vi "Test Comm Multi.vi"() -> ()   [LabVIEW 2021]
uses:
  ChannelCommon/typedef/FIFO Config.ctl
  ChannelCommon/ChannelCommon.lvlib
  CIFChannels/Typedef/Direction.ctl
  CIFChannels/CIFChannels.lvclass
  ChannelCommon/typedef/TimeStamps.ctl
  FIFO_U8_Multi/CIF_Fifo_U8_Multi.lvclass
  ChannelCommon/typedef/New FIFO Instance Configuration.ctl
  FIFO_U8/CIF_NIChn_Fifo_U8.lvclass
  D:/dev/Packages/Channel_Manager/src/CIF_NIChn/FIFO_U8/CIF_NIChn_Fifo_U8.lvclass
  D:/dev/Packages/Channel_Manager/src/CIF_NIChn/NIChn/CIF_NIChn.lvclass
  D:/dev/Packages/Channel_Manager/src/CIFChannels/CIFChannels.lvclass
  D:/dev/Packages/Channel_Manager/src/CIF_NIChn/FIFO_U8_Multi/CIF_Fifo_U8_Multi.lvclass
  CIF_Fifo_Raw.lvclass
  D:/dev/Packages/Channel_Manager/src/CIF_NIChn/FIFO_RAW_Multi/CIF_Fifo_Raw.lvclass
panel:
  out "status":string
  out "pass":bool
  out "error out":errorcluster
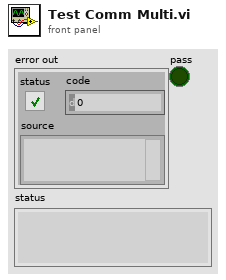
[diagram p1: front panel]
types:
  T1 = typedef "CIFChannels.lvclass/Direction.ctl" = enum16{"Publisher", "Subscriber"}
  T2 = typedef "ChannelCommon.lvlib/New FIFO Instance Configuration.ctl" = cluster{"Primary":bool, "Backpressure":bool, "Message/FIFO Override":u32}
  T3 = typedef "ChannelCommon.lvlib/TimeStamps.ctl" = cluster{"ClockID":u8, "T0":i64, "T_Out":i64}
  T4 = typedef "ChannelCommon.lvlib/FIFO Config.ctl" = cluster{"Max Bytes/Msg":u64, "Max Msg/FIFO":u64, "Flags":u64}
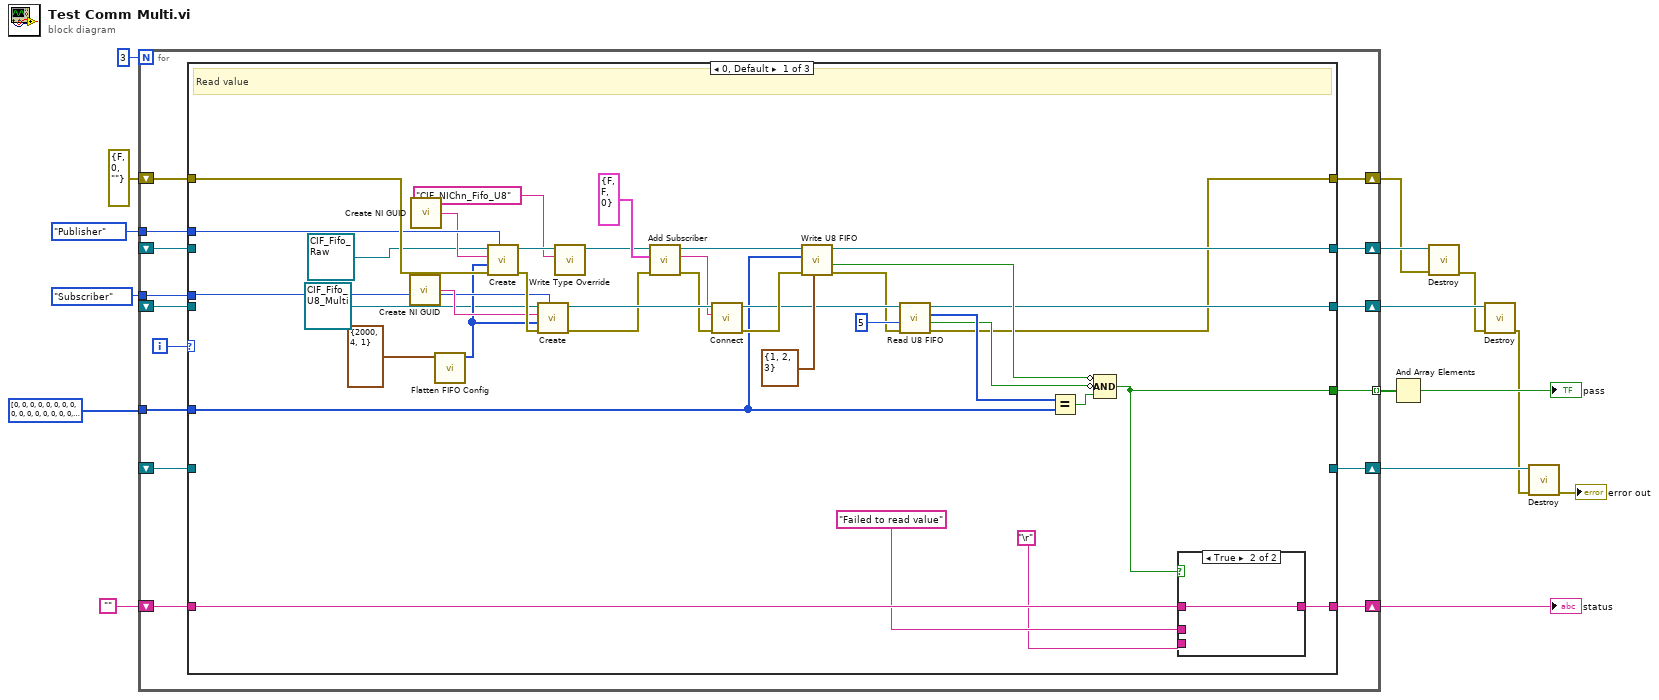
[diagram p0: block diagram]
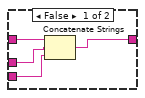
[diagram p2: hidden frame]
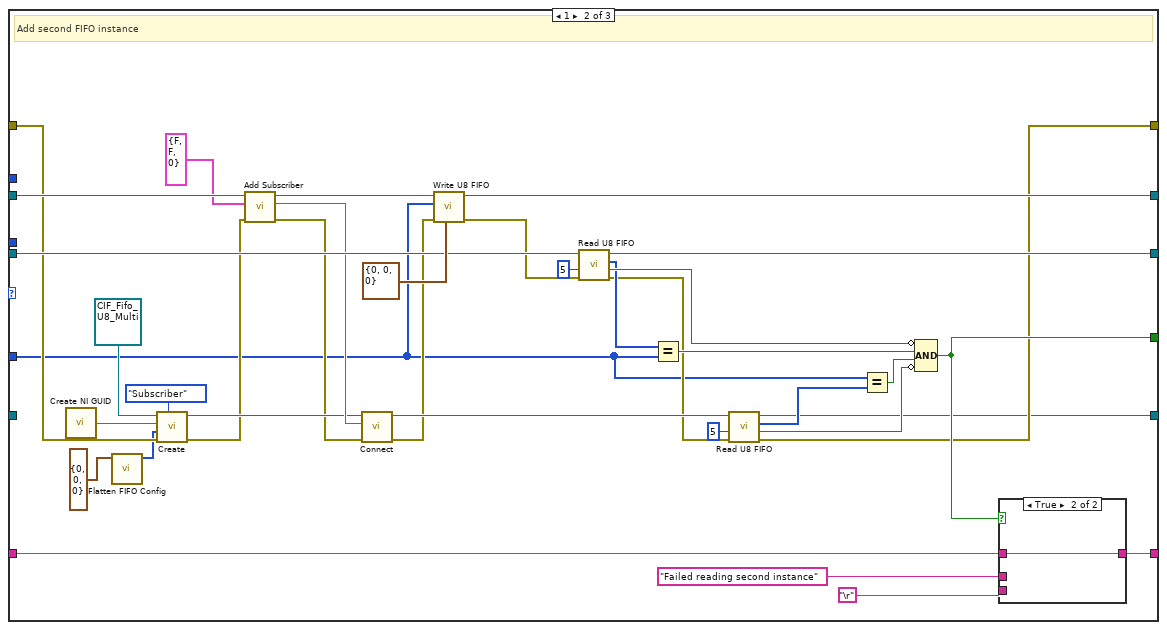
[diagram p3: hidden frame]
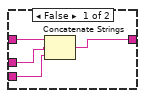
[diagram p4: hidden frame]
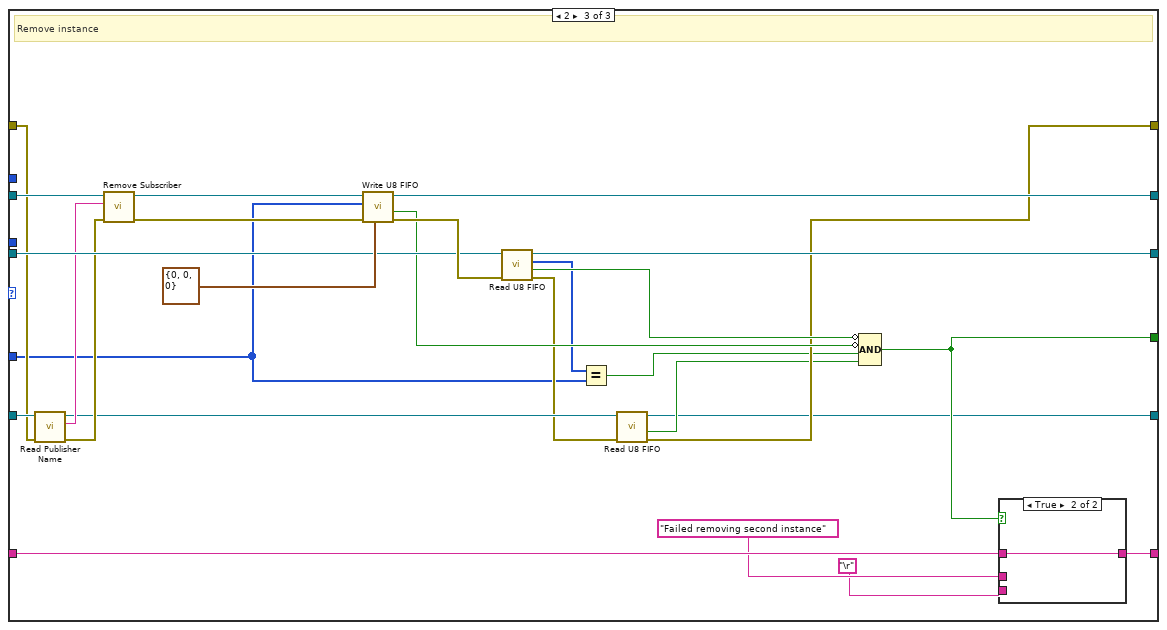
[diagram p5: hidden frame]
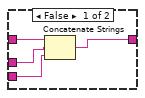
[diagram p6: hidden frame]
diagram:
  n1 = for {
    N: 3 -> [_]
    tunnel: [w31] -> w16 mode=indexing
    shift-right: [w22] -> w6
    shift-left: errorcluster {"status"=FALSE, "code"=0, "source"=""} ("error out") -> [w30]
    shift-right: [w27] -> w12
    shift-left: "" -> [w28]
    tunnel: Direction."Subscriber" ("Direction") -> [w26]
    tunnel: Direction."Publisher" ("Direction") -> [w25]
    shift-right: [w24] -> w8
    shift-left: _ -> [w20]
    shift-right: [w23] -> w7
    shift-left: _ -> [w21]
    tunnel: u8[] [0, 0, 0, 0, 0, 0, 0, 0, 0, 0, 0, 0, 0, 0, 0, 0, 0, 0, 0, 0, 0, 0, 0, 0, 0, 0, 0, 0, 0, 0, 0, 0, 0, 0, 0, 0, 0, 0, 0, 0, 0, 0, 0, 0, 0, 0, 0, 0, 0, 0, 0, 0, 0, 0, 0, 0, 0, 0, 0, 0, 0, 0, 0, 0, 0, 0, 0, 0, 0, 0, 0, 0, 0, 0, 0, 0, 0, 0, 0, 0, 0, 0, 0, 0, 0, 0, 0, 0, 0, 0, 0, 0, 0, 0, 0, 0, 0, 0, 0, 0, 0, 0, 0, 0, 0, 0, 0, 0, 0, 0, 0, 0, 0, 0, 0, 0, 0, 0, 0, 0, 0, 0, 0, 0, 0, 0, 0, 0, 0, 0, 0, 0, 0, 0, 0, 0, 0, 0, 0, 0, 0, 0, 0, 0, 0, 0, 0, 0, 0, 0, 0, 0, 0, 0, 0, 0, 0, 0, 0, 0, 0, 0, 0, 0, 0, 0, 0, 0, 0, 0, 0, 0, 0, 0, 0, 0, 0, 0, 0, 0, 0, 0, 0, 0, 0, 0, 0, 0, 0, 0, 0, 0, 0, 0, 0, 0, 0, 0, 0, 0, 0, 0, 0, 0, 0, 0, 0, 0, 0, 0, 0, 0, 0, 0, 0, 0, 0, 0, 0, 0, 0, 0, 0, 0, 0, 0, 0, 0, 0, 0, 0, 0, 0, 0, 0, 0, 0, 0, 0, 0, 0, 0, 0, 0, 0, 0, 0, 0, 0, 0, 0, 0, 0, 0, 0, 0, 0, 0, 0, 0, 0, 0, 0, 0, 0, 0, 0, 0, 0, 0, 0, 0, 0, 0, 0, 0, 0, 0, 0, 0, 0, 0, 0, 0, 0, 0, 0, 0, 0, 0, 0, 0, 0, 0, 0, 0, 0, 0, 0, 0, 0, 0, 0, 0, 0, 0, 0, 0, 0, 0, 0, 0, 0, 0, 0, 0, 0, 0, 0, 0, 0, 0, 0, 0, 0, 0, 0, 0, 0, 0, 0, 0, 0, 0, 0, 0, 0, 0, 0, 0, 0, 0, 0, 0, 0, 0, 0, 0, 0, 0, 0, 0, 0, 0, 0, 0, 0, 0, 0, 0, 0, 0, 0, 0, 0, 0, 0, 0, 0, 0, 0, 0, 0, 0, 0, 0, 0, 0, 0, 0, 0, 0, 0, 0, 0, 0, 0, 0, 0, 0, 0, 0, 0, 0, 0, 0, 0, 0, 0, 0, 0, 0, 0, 0, 0, 0, 0, 0, 0, 0, 0, 0, 0, 0, 0, 0, 0, 0, 0, 0, 0, 0, 0, 0, 0, 0, 0, 0, 0, 0, 0, 0, 0, 0, 0, 0, 0, 0, 0, 0, 0, 0, 0, 0, 0, 0, 0, 0, 0, 0, 0, 0, 0, 0, 0, 0, 0, 0, 0, 0, 0, 0, 0, 0, 0, 0, 0, 0, 0, 0, 0, 0, 0, 0, 0, 0, 0, 0, 0, 0, 0, 0, 0, 0, 0, 0, 0, 0, 0, 0, 0, 0, 0, 0, 0, 0, 0, 0, 0, 0, 0, 0, 0, 0, 0, 0, 0, 0, 0, 0, 0, 0, 0, 0, 0, 0, 0, 0, 0, 0, 0, 0, 0, 0, 0, 0, 0, 0, 0, 0, 0, 0, 0, 0, 0, 0, 0, 0, 0, 0, 0, 0, 0, 0, 0, 0, 0, 0, 0, 0, 0, 0, 0, 0, 0, 0, 0, 0, 0, 0, 0, 0, 0, 0, 0, 0, 0, 0, 0, 0, 0, 0, 0, 0, 0, 0, 0, 0, 0, 0, 0, 0, 0, 0, 0, 0, 0, 0, 0, 0, 0, 0, 0, 0, 0, 0, 0, 0, 0, 0, 0, 0, 0, 0, 0, 0, 0, 0, 0, 0, 0, 0, 0, 0, 0, 0, 0, 0, 0, 0, 0, 0, 0, 0, 0, 0, 0, 0, 0, 0, 0, 0, 0, 0, 0, 0, 0, 0, 0, 0, 0, 0, 0, 0, 0, 0, 0, 0, 0, 0, 0, 0, 0, 0, 0, 0, 0, 0, 0, 0, 0, 0, 0, 0, 0, 0, 0, 0, 0, 0, 0, 0, 0, 0, 0, 0, 0, 0, 0, 0, 0, 0, 0, 0, 0, 0, 0, 0, 0, 0, 0, 0, 0, 0, 0, 0, 0, 0, 0, 0, 0, 0, 0, 0, 0, 0, 0, 0, 0, 0, 0, 0, 0, 0, 0, 0, 0, 0, 0, 0, 0, 0, 0, 0, 0, 0, 0, 0, 0, 0, 0, 0, 0, 0, 0, 0, 0, 0, 0, 0, 0, 0, 0, 0, 0, 0, 0, 0, 0, 0, 0, 0, 0, 0, 0, 0, 0, 0, 0, 0, 0, 0, 0, 0, 0, 0, 0, 0, 0, 0, 0, 0, 0, 0, 0, 0, 0, 0, 0, 0, 0, 0, 0, 0, 0, 0, 0, 0, 0, 0, 0, 0, 0, 0, 0, 0, 0, 0, 0, 0, 0, 0, 0, 0, 0, 0, 0, 0, 0, 0, 0, 0, 0, 0, 0, 0, 0, 0, 0, 0, 0, 0, 0, 0, 0, 0, 0, 0, 0, 0, 0, 0, 0, 0, 0, 0, 0, 0, 0, 0, 0, 0, 0, 0, 0, 0, 0, 0, 0, 0, 0, 0, 0, 0, 0, 0, 0, 0, 0, 0, 0, 0, 0, 0, 0, 0, 0, 0, 0, 0, 0, 0, 0, 0, 0, 0, 0, 0, 0, 0, 0, 0, 0, 0, 0, 0, 0, 0, 0, 0, 0, 0, 0, 0, 0, 0, 0, 0, 0, 0, 0, 0, 0, 0, 0, 0, 0, 0, 0, 0, 0, 0, 0, 0, 0, 0, 0, 0, 0, 0, 0, 0, 0, 0, 0, 0, 0, 0, 0, 0, 0, 0, 0, 0, 0, 0, 0, 0, 0, 0, 0, 0, 0, 0, 0, 0, 0, 0, 0, 0, 0, 0, 0, 0, 0, 0, 0, 0, 0, 0, 0, 0, 0, 0, 0, 0, 0, 0, 0, 0, 0, 0, 0, 0, 0, 0, 0, 0, 0, 0, 0, 0, 0, 0, 0, 0, 0, 0, 0, 0, 0, 0, 0, 0, 0, 0, 0, 0, 0, 0, 1] ("Data in") -> [w19]
    shift-right: [w17] -> w4
    shift-left: _ -> [w18]
    i -> [w29]
    n2 = case shown="0, Default" w29 {
      tunnel: [w63 w106 w136] -> w31
      tunnel: w30 -> [w61 w89 w129]
      tunnel: [w44 w79 w121] -> w22
      tunnel: w28 -> [w68 w110 w142]
      tunnel: [w67 w109 w141] -> w27
      tunnel: w26 -> [w59 _ _]
      tunnel: w25 -> [w58 _ _]
      tunnel: [w46 w80 w133] -> w24
      tunnel: [w51 w98 w124] -> w23
      tunnel: w21 -> [_ w97 w132]
      tunnel: w20 -> [_ w99 w134]
      tunnel: w19 -> [w37 w78 w117]
      tunnel: w18 -> [_ _ w130]
      tunnel: [_ w74 w116] -> w17
      frame 0, Default {
        # "Read value"
        n3 = call <vilib>:"Create NI GUID.vi"() -> ("NI GUID"=w60:string)
        n4 = call <vilib>:"Create NI GUID.vi"() -> ("NI GUID"=w56:string)
        n5 = call "Flatten FIFO Config.vi"("FIFO Config in"=T4 {"Max Bytes/Msg"=2000, "Max Msg/FIFO"=4, "Flags"=1}) -> ("Flattened FIFO Config"=w54:u8[])  [unwired: 10 in]
        n6 = call-dynamic "Create.vi"("Direction"=w58, "error in (no error)"=w61, "Custom Config Data"=w54, "Name"=w56, "CIF_Fifo_Raw_Multi in"=refnum<class "CIF_Fifo_Raw.lvclass"> refnum ("CIF_Fifo_Raw_Multi.lvclass")) -> ("error out"=w62:errorcluster, "CIF_Fifo_Raw_Multi out"=w34:refnum<class "CIF_Fifo_Raw.lvclass">)  [unwired: 5 in]
        n7 = call-dynamic "Create.vi"("Direction"=w59, "error in (no error)"=w62, "Custom Config Data"=w54, "Name"=w60, "CIF_Fifo_U8 in"=refnum<class "CIF_Fifo_U8_Multi.lvclass"> refnum ("CIF_DAQ_DVR_Multi.lvclass")) -> ("error out"=w40:errorcluster, "CIF_Fifo_U8 out"=w55:refnum<class "CIF_Fifo_U8_Multi.lvclass">)  [unwired: 5 in]
        n8 = call "Write Type Override.vi"("Type Override"="CIF_NIChn_Fifo_U8", "CIF_Fifo_Raw_Multi in"=w34) -> ("CIF_Fifo_Raw_Multi out"=w33:refnum<class "CIF_Fifo_Raw.lvclass">)  [unwired: 8 in, 1 out]
        n9 = call-dynamic "Add Subscriber.vi"("error in (no error)"=w40, "New FIFO Instance Config"=T2 {"Primary"=FALSE, "Backpressure"=FALSE, "Message/FIFO Override"=0}, "CIF_Fifo_Raw_Multi in"=w33) -> ("error out"=w39:errorcluster, "New Publisher"=w41:string, "CIF_Fifo_Raw_Multi out"=w42:refnum<class "CIF_Fifo_Raw.lvclass">)  [unwired: 6 in]
        n10 = call-dynamic "Connect.vi"("error in (no error)"=w39, "Connection Name"=w41, "CIFTag in"=w55) -> ("error out"=w53:errorcluster, "CIFTag out"=w49:refnum<class "CIF_Fifo_U8_Multi.lvclass">)  [unwired: 7 in]
        n11 = call-dynamic "Write U8 FIFO.vi"("FIFO Timestamps"=T3 {"ClockID"=1, "T0"=2, "T_Out"=3}, "error in (no error)"=w53, "Data in"=w37, "CIF_Fifo_U8 in"=w42) -> ("error out"=w36:errorcluster, "timed out?"=w50:bool, "CIF_Fifo_U8 out"=w51:refnum<class "CIF_Fifo_Raw.lvclass">)  [unwired: 4 in, 1 out]
        n12 = call-dynamic "Read U8 FIFO.vi"("error in (no error)"=w36, "Timeout (ms)"=5, "CIFFIFO in"=w49) -> ("error out"=w44:errorcluster, "timed out?"=w45:bool, "Data out"=w47:u8[], "CIFFIFO out"=w46:refnum<class "CIF_Fifo_U8_Multi.lvclass">)  [unwired: 4 in, 1 out]
        n13 = Equal?(x=w47, y=w37) -> (x = y?=w64:bool)
        n14 = Compound Arithmetic op=AND(invert w50, invert w45, w64) -> (w63:bool)
        n15 = case shown="True" w63 {
          tunnel: w68 -> [w72 w73]
          tunnel: [w69 w73] -> w67
          tunnel: "Failed to read value" -> [w71 _]
          tunnel: "\r" -> [w70 _]
          frame False {
            n16 = Concatenate Strings(w72, w71, w70) -> (w69:string)
          }
          frame True {
          }
        }
      }
      frame 1 {
        # "Add second FIFO instance"
        n17 = call <vilib>:"Create NI GUID.vi"() -> ("NI GUID"=w94:string)
        n18 = call "Flatten FIFO Config.vi"("FIFO Config in"=T4 {"Max Bytes/Msg"=0, "Max Msg/FIFO"=0, "Flags"=0}) -> ("Flattened FIFO Config"=w88:u8[])  [unwired: 10 in]
        n19 = call-dynamic "Create.vi"("Direction"=Direction."Subscriber", "error in (no error)"=w89, "Custom Config Data"=w88, "Name"=w94, "CIF_Fifo_U8 in"=refnum<class "CIF_Fifo_U8_Multi.lvclass"> refnum ("CIF_DAQ_DVR_Multi.lvclass")) -> ("error out"=w90:errorcluster, "CIF_Fifo_U8 out"=w92:refnum<class "CIF_Fifo_U8_Multi.lvclass">)  [unwired: 5 in]
        n20 = call-dynamic "Add Subscriber.vi"("error in (no error)"=w90, "New FIFO Instance Config"=T2 {"Primary"=FALSE, "Backpressure"=FALSE, "Message/FIFO Override"=0}, "CIF_Fifo_U8 in"=w97) -> ("error out"=w91:errorcluster, "New Publisher"=w93:string, "CIF_Fifo_U8 out"=w96:refnum<class "CIF_Fifo_U8_Multi.lvclass">)  [unwired: 6 in]
        n21 = call-dynamic "Connect.vi"("error in (no error)"=w91, "Connection Name"=w93, "CIFTag in"=w92) -> ("error out"=w83:errorcluster, "CIFTag out"=w84:refnum<class "CIF_Fifo_U8_Multi.lvclass">)  [unwired: 7 in]
        n22 = call-dynamic "Write U8 FIFO.vi"("FIFO Timestamps"=T3 {"ClockID"=0, "T0"=0, "T_Out"=0}, "error in (no error)"=w83, "Data in"=w78, "CIF_Fifo_U8 in"=w96) -> ("error out"=w77:errorcluster, "CIF_Fifo_U8 out"=w98:refnum<class "CIF_Fifo_U8_Multi.lvclass">)  [unwired: 4 in, 2 out]
        n23 = call-dynamic "Read U8 FIFO.vi"("error in (no error)"=w77, "Timeout (ms)"=5, "CIFFIFO in"=w99) -> ("error out"=w81:errorcluster, "timed out?"=w102:bool, "Data out"=w101:u8[], "CIFFIFO out"=w80:refnum<class "CIF_NIChn_Fifo_U8.lvclass">)  [unwired: 4 in, 1 out]
        n24 = Equal?(x=w101, y=w78) -> (x = y?=w104:bool)
        n25 = call-dynamic "Read U8 FIFO.vi"("error in (no error)"=w81, "Timeout (ms)"=5, "CIFFIFO in"=w84) -> ("error out"=w79:errorcluster, "timed out?"=w75:bool, "Data out"=w82:u8[], "CIFFIFO out"=w74:refnum<class "CIF_Fifo_U8_Multi.lvclass">)  [unwired: 4 in, 1 out]
        n26 = Equal?(x=w78, y=w82) -> (x = y?=w105:bool)
        n27 = Compound Arithmetic op=AND(invert w102, w104, w105, invert w75) -> (w106:bool)
        n28 = case shown="True" w106 {
          tunnel: w110 -> [w114 w115]
          tunnel: [w111 w115] -> w109
          tunnel: "Failed reading second instance" -> [w113 _]
          tunnel: "\r" -> [w112 _]
          frame False {
            n29 = Concatenate Strings(w114, w113, w112) -> (w111:string)
          }
          frame True {
          }
        }
      }
      frame 2 {
        # "Remove instance"
        n30 = call "Read Publisher Name.vi"("error in (no error)"=w129, "CIFChannels in"=w130) -> ("error out"=w126:errorcluster, "Publisher Name"=w128:string, "CIFChannels out"=w123:refnum<class "CIF_Fifo_U8_Multi.lvclass">)  [unwired: 7 in]
        n31 = call-dynamic "Remove Subscriber.vi"("error in (no error)"=w126, "Publisher to Remove"=w128, "CIF_Fifo_U8 in"=w132) -> ("error out"=w127:errorcluster, "CIF_Fifo_U8 out"=w131:refnum<class "CIF_Fifo_U8_Multi.lvclass">)  [unwired: 7 in]
        n32 = call-dynamic "Write U8 FIFO.vi"("FIFO Timestamps"=T3 {"ClockID"=0, "T0"=0, "T_Out"=0}, "error in (no error)"=w127, "Data in"=w117, "CIF_Fifo_U8 in"=w131) -> ("error out"=w138:errorcluster, "timed out?"=w125:bool, "CIF_Fifo_U8 out"=w124:refnum<class "CIF_Fifo_U8_Multi.lvclass">)  [unwired: 4 in, 1 out]
        n33 = call-dynamic "Read U8 FIFO.vi"("error in (no error)"=w138, "CIFFIFO in"=w134) -> ("error out"=w122:errorcluster, "timed out?"=w137:bool, "Data out"=w120:u8[], "CIFFIFO out"=w133:refnum<class "CIF_NIChn_Fifo_U8.lvclass">)  [unwired: 5 in, 1 out]
        n34 = Equal?(x=w120, y=w117) -> (x = y?=w119:bool)
        n35 = call-dynamic "Read U8 FIFO.vi"("error in (no error)"=w122, "CIFFIFO in"=w123) -> ("error out"=w121:errorcluster, "timed out?"=w118:bool, "CIFFIFO out"=w116:refnum<class "CIF_Fifo_U8_Multi.lvclass">)  [unwired: 5 in, 2 out]
        n36 = Compound Arithmetic op=AND(invert w137, invert w125, w119, w118) -> (w136:bool)
        n37 = case shown="True" w136 {
          tunnel: w142 -> [w146 w147]
          tunnel: [w143 w147] -> w141
          tunnel: "Failed removing second instance" -> [w145 _]
          tunnel: "\r" -> [w144 _]
          frame False {
            n38 = Concatenate Strings(w146, w145, w144) -> (w143:string)
          }
          frame True {
          }
        }
      }
    }
  }
  "status" <- w12
  n39 = And Array Elements(Boolean array=w16) -> (logical AND=→"pass":bool)
  n40 = call-dynamic "Destroy.vi"("error in (no error)"=w6, "CIF_Fifo_U8 in"=w7) -> ("error out"=w5:errorcluster)  [unwired: 8 in, 1 out]
  n41 = call-dynamic "Destroy.vi"("error in (no error)"=w5, "CIFFIFO in"=w8) -> ("error out"=w3:errorcluster)  [unwired: 8 in, 1 out]
  n42 = call-dynamic "Destroy.vi"("error in (no error)"=w3, "CIF_Fifo_U8 in"=w4) -> ("error out"=→"error out":errorcluster)  [unwired: 8 in, 1 out]
